vi "Read magnet system configuration.vi"(8 "error in (no error)":errorcluster, 11 "MAG config file path":path) -> (0 "error out":errorcluster, 3 "Magnet Constantsout":T1={"Switch resistant [K]"=5.0, "Switch superconducting [K]"=4.0, "First stage critical temperature [K]"=50.0, "Second stage critical temperature [K]"=5.0, "Inner magnet critical temperature [K]"=6.0, "Outer magnet critical temperature [K]"=5.0, "Field Constant [T/A]"=0.14911, "Maximum Current [A]"=107.3, "Maximum field [T]"=16.0, "Maximum source ramp [A/s]"=0.5, "Source precision [T]"=2e-05, "Ramp limits [A/s]"=[0.0506, 0.038, 0.0285, 0.0213, 0.0104], "Field limits [T]"=[3.0, 9.6, 13.3, 15.5, 16.0], "SMS"="COM3", "LSC218"="COM1"}, 4 "file path out":path)   [LabVIEW 2022 SP3]
doc: "Reads an INI file with magnet configuration data, for example port names and maximum ramp/field constants.\nConsiderable build-in function: searching for SMS serial port"
uses:
  Subsystem modules/Magnet module/ctl/Magnet config constants.ctl
  <userlib>/_OpenG.lib/variantconfig/variantconfig.llb/openg_variant_configuration_file.lvlib
  <vilib>/Utility/config.llb/NI_LVConfig.lvlib
  Subsystem modules/Magnet module/Magnet module.lvlib
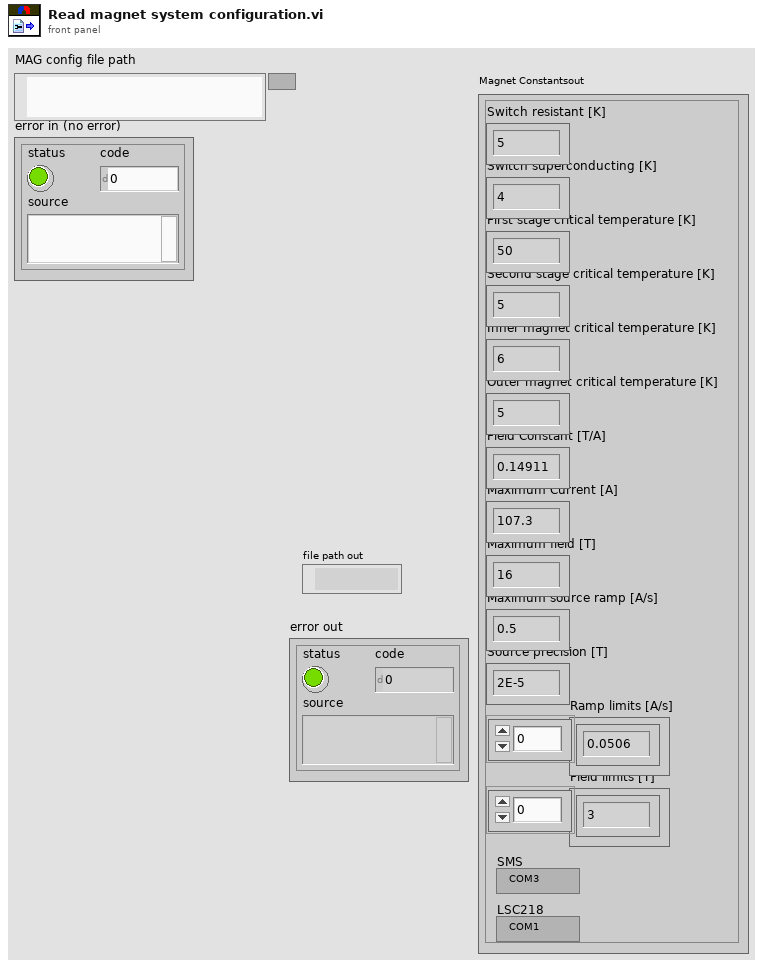
[diagram p1: front panel]
types:
  T1 = typedef "Magnet module.lvlib/Magnet config constants.ctl" = cluster{"Switch resistant [K]":dbl, "Switch superconducting [K]":dbl, "First stage critical temperature [K]":dbl, "Second stage critical temperature [K]":dbl, "Inner magnet critical temperature [K]":dbl, "Outer magnet critical temperature [K]":dbl, "Field Constant [T/A]":dbl, "Maximum Current [A]":dbl, "Maximum field [T]":dbl, "Maximum source ramp [A/s]":dbl, "Source precision [T]":dbl, "Ramp limits [A/s]":dbl[], "Field limits [T]":dbl[], "SMS":refnum<visa-resource-name>, "LSC218":refnum<visa-resource-name>}
  T2 = typedef "NI_LVConfig.lvlib/Config Data RefNum.ctl" = refnum<k1>
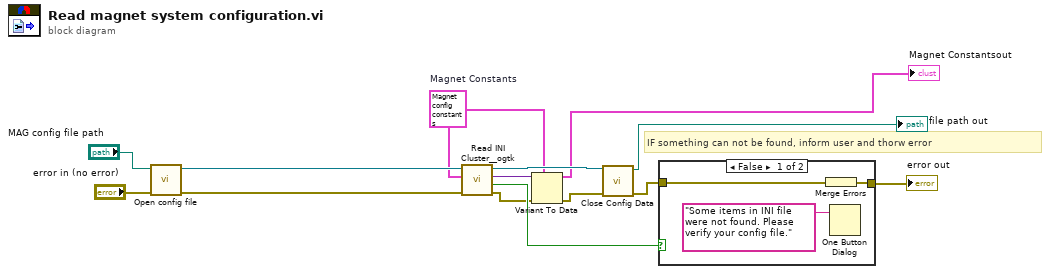
[diagram p0: block diagram]
diagram:
  w2 = T1 {"Switch resistant [K]"=5.0, "Switch superconducting [K]"=4.0, "First stage critical temperature [K]"=50.0, "Second stage critical temperature [K]"=5.0, "Inner magnet critical temperature [K]"=6.0, "Outer magnet critical temperature [K]"=5.0, "Field Constant [T/A]"=0.14911, "Maximum Current [A]"=107.3, "Maximum field [T]"=16.0, "Maximum source ramp [A/s]"=0.5, "Source precision [T]"=2e-05, "Ramp limits [A/s]"=[0.0506, 0.038, 0.0285, 0.0213, 0.0104], "Field limits [T]"=[3.0, 9.6, 13.3, 15.5, 16.0], "SMS"="COM3", "LSC218"="COM1"}  # Magnet Constants
  # "IF something can not be found, inform user and thorw error"
  n1 = call "Open config file.vi"("error in (no error)"="error in (no error)", "MAG config file path"="MAG config file path") -> ("error out"=w3:errorcluster, "Refnum out"=w4:T2)  [unwired: 6 in, 2 out]
  n2 = call <userlib>:"Read INI Cluster__ogtk.vi"("error in (no error)"=w3, "INI Fomatted Cluster Type"=w2, "refnum"=w4) -> ("error out"=w9:errorcluster, "all found?"=w13:bool, "INI Fomatted Cluster"=w14:variant, "dup refnum"=w12:T2)  [unwired: 4 in, 1 out]
  n3 = Variant To Data(error in=w9, type=w2, Variant=w14) -> (data=→"Magnet Constantsout":T1, error out=w8:errorcluster)
  n4 = call <vilib>:"Close Config Data.vi"("error in (no error)"=w8, "refnum"=w12) -> ("error out"=w11:errorcluster, "file path"=→"file path out":path)  [unwired: 8 in]
  n5 = case shown="False" w13 {
    tunnel: [w15 w18] -> w10
    tunnel: w11 -> [w16 w18]
    frame False {
      n6 = Merge Errors(w16) -> (w15:errorcluster)
      n7 = One Button Dialog(message="Some items in INI file were not found. Please verify your config file.") -> ()  [unwired: 1 in, 1 out]
    }
    frame True {
    }
  }
  "error out" <- w10
